vi "dataAcq_channel.vi"(8 "error in (no error)":errorcluster, 11 "Thorlabs_OSA_64 in":refnum<class "OSA.lvclass">) -> (0 "error out":errorcluster, 3 "Thorlabs_OSA_64 out":refnum<class "OSA.lvclass">)   [LabVIEW 2010, in "OSA.lvclass"]
uses:
  OSA.lvclass
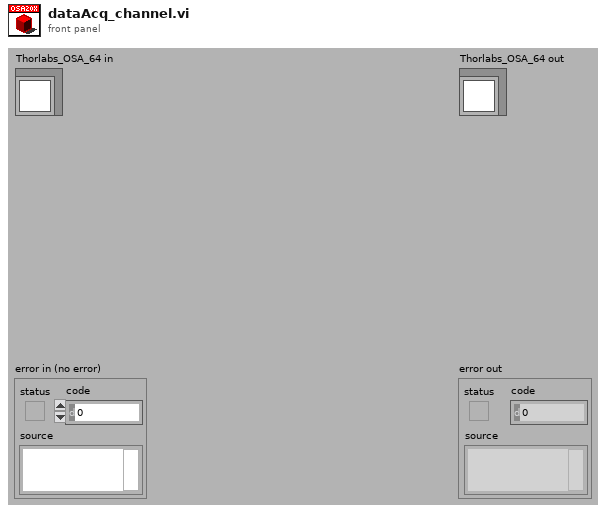
[diagram p1: front panel]
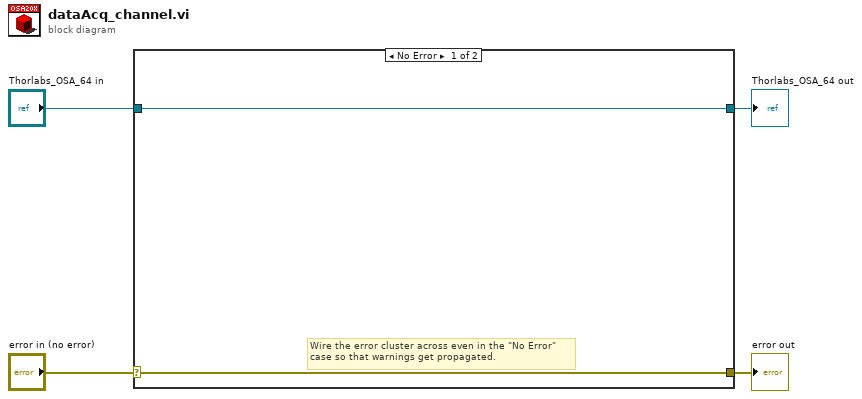
[diagram p0: block diagram]
diagram:
  n1 = case shown="No Error" "error in (no error)" {
    selector: "error in (no error)" -> [w5 w8]
    tunnel: [w5 w8] -> w3
    tunnel: [w6 w7] -> w1
    tunnel: "Thorlabs_OSA_64 in" -> [w6 w7]
    frame No Error {
      # "Wire the error cluster across even in the \"No Error\"\ncase so that warnings get propagated."
    }
    frame Error {
    }
  }
  "error out" <- w3
  "Thorlabs_OSA_64 out" <- w1
